vi "Write frozenColumn.vi"(8 "error in (no error)":errorcluster, 10 "frozenColumn":i32, 11 "DataGridView in":refnum<class "DataGridView.lvclass">) -> (0 "error out":errorcluster, 3 "DataGridView out":refnum<class "DataGridView.lvclass">)   [LabVIEW 2013, in "DataGrid.lvlib" / "DataGridView.lvclass"]
uses:
  DataGridView.lvclass
  System.Windows.Forms
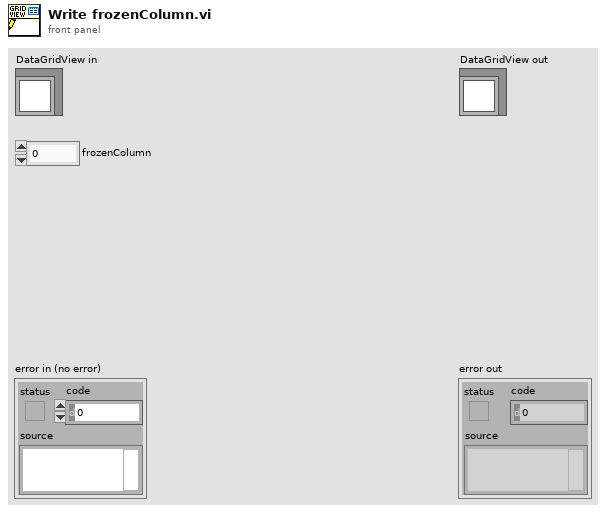
[diagram p1: front panel]
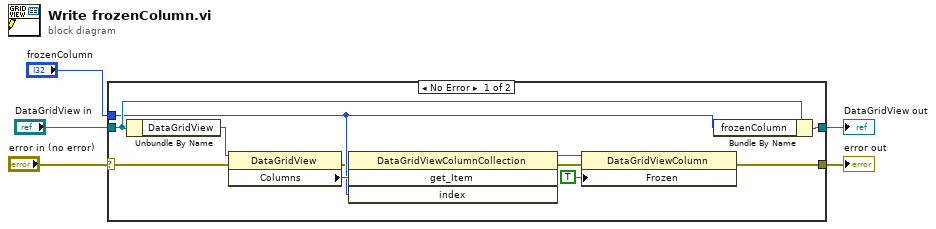
[diagram p0: block diagram]
diagram:
  n1 = case shown="No Error" "error in (no error)" {
    selector: "error in (no error)" -> [w7 w17]
    tunnel: [w6 w17] -> w4
    tunnel: [w16 w18] -> w2
    tunnel: "DataGridView in" -> [w15 w18]
    tunnel: "frozenColumn" -> [w12 _]
    frame No Error {
      n2 = Unbundle By Name(w15) -> ("DataGridView"=w14:refnum<k24>)
      n3 = property class="DataGridView"(reference=w14, error in=w7) -> (error out=w9:errorcluster, "Columns"=w13:refnum<k24>)  [unwired: 1 out]
      n4 = invoke class="DataGridViewColumnCollection" method="get_Item"(reference=w13, error in=w9, "index"=w12) -> (error out=w8:errorcluster, "get_Item"=w11:refnum<k24>)  [unwired: 1 in, 2 out]
      n5 = property class="DataGridViewColumn"(reference=w11, error in=w8, "Frozen"=TRUE) -> (error out=w6:errorcluster)  [unwired: 1 out]
      n6 = Bundle By Name(cluster=w15, "frozenColumn"=w12) -> (w16:refnum<class "DataGridView.lvclass">)
    }
    frame Error {
    }
  }
  "error out" <- w4
  "DataGridView out" <- w2
